vi "CSV Read Config.vi"(8 "error in (no error)":errorcluster, 11 "CSV Section Name":string) -> (0 "error out":errorcluster, 3 "Header":string)   [LabVIEW 2025]
uses:
  <vilib>/Utility/config.llb/NI_LVConfig.lvlib
  <vilib>/Utility/config.llb/Read Key (String).vi
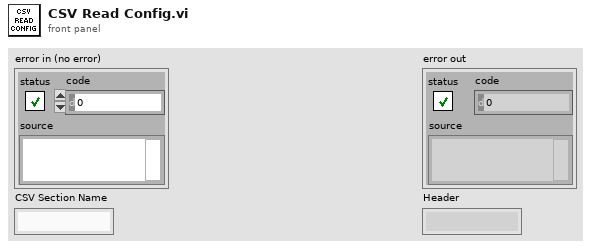
[diagram p1: front panel]
types:
  T1 = typedef "NI_LVConfig.lvlib/Config Data RefNum.ctl" = refnum<k1>
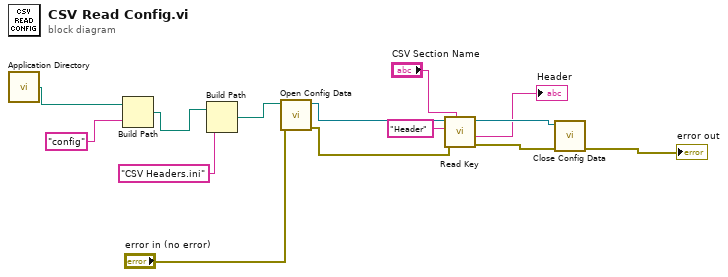
[diagram p0: block diagram]
diagram:
  n1 = call <vilib>:"Application Directory.vi"() -> ("Application Directory"=w14:path)
  n2 = Build Path(base path=w14, name or relative path="config" ("regular expression")) -> (appended path=w12:path)
  n3 = Build Path(base path=w12, name or relative path="CSV Headers.ini" ("regular expression")) -> (appended path=w11:path)
  n4 = call <vilib>:"Open Config Data.vi"("error in (no error)"="error in (no error)", "configuration file path"=w11) -> ("error out"=w6:errorcluster, "refnum"=w10:T1)  [unwired: 7 in, 1 out]
  n5 = call-poly <vilib>:"Read Key.vi"("section"="CSV Section Name", "error in (no error)"=w6, "key"="Header", "refnum"=w10) -> ("error out"=w5:errorcluster, "value"=→"Header":string, "refnum out"=w8:T1)  [unwired: 4 in, 1 out]
  n6 = call <vilib>:"Close Config Data.vi"("error in (no error)"=w5, "refnum"=w8) -> ("error out"=→"error out":errorcluster)  [unwired: 8 in, 1 out]
